vi "GVSGraph XY Window.vi"() -> ()   [LabVIEW 2013]
panel:
  out "StateOut":bool=TRUE
  in  "GraphType":string
  out "Event Name":string
  out "Queue Name":string
  out "Title Name":string
  out "Graph Number":i32
  out "XY Graph":cluster{"X":dbl, "Y":dbl}[](graph)
  in  "Parent_Index":i32
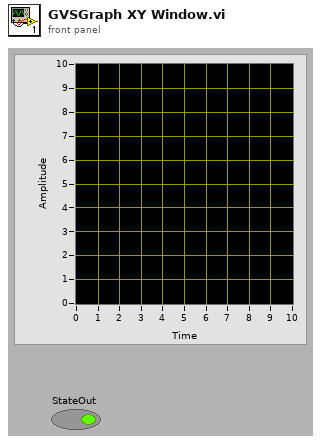
[diagram p1: front panel]
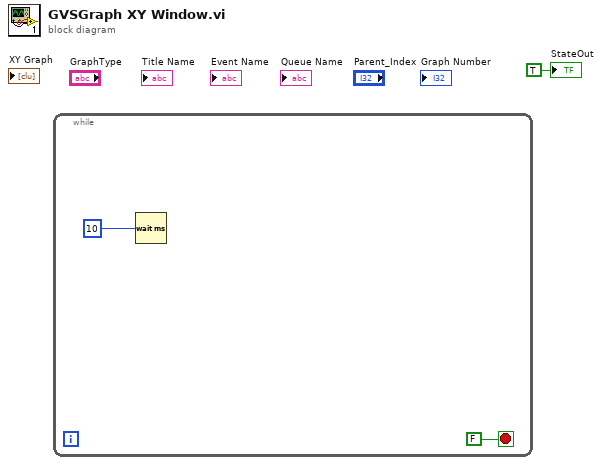
[diagram p0: block diagram]
diagram:
  n1 = while {
    stop <- FALSE stop-if-true
    n2 = Wait (ms)(milliseconds to wait=u32 10) -> ()  [unwired: 1 out]
  }
  "StateOut" <- TRUE ("StateOut")
